vi "zadanie_1.vi"() -> ()   [LabVIEW 2020]
panel:
  out "Array 2":i32[](array[numeric])
  out "Array":i32[](array[numeric])
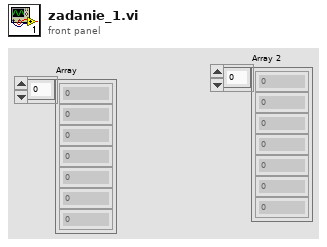
[diagram p1: front panel]
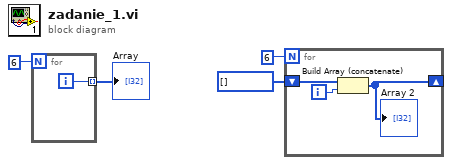
[diagram p0: block diagram]
diagram:
  n1 = for {
    N: 6 -> [_]
    tunnel: [w5] -> w3 mode=indexing
    i -> [w5]
  }
  "Array" <- w3
  n2 = for {
    N: 6 -> [_]
    shift-right: [w6] -> _
    shift-left: i32[] [] ("Array") -> [w7]
    i -> [w8]
    n3 = Build Array (concatenate)(w7, w8) -> (w6:i32[])
    "Array 2" <- w6
  }
